vi "Updating Existing Tree from XML.vi"() -> ()   [LabVIEW 2017, in "Tree API.lvlib" / "Tree.lvclass"]
uses:
  Tree.lvclass
  API/Set Attributes Tree Data.vi
  Data Types/Float/To Float Tree Data.vi
  Data Types/Float/Flt.lvclass
  Data Types/Bool/To Bool Tree Data.vi
  Data Types/Bool/Bool.lvclass
panel:
  in  "Setpoint 2":dbl=2.0 format="%#_13g"
  in  "Setpoint 1":dbl=-1.0 format="%#_13g"
  in  "Run HW":bool=TRUE
  in  "Enable CFG":bool
  out "XML On RT":string="<Received_Configuration>\n<Enable_CFG Type=\"Bool\">\r\nFALSE\r\n</Enable_CFG>\r\n<Run_HW Type=\"Bool\">\r\nTRUE\r\n</Run_HW>\r\n<Setpoint_1 Type=\"Flt\">\r\n-1\r\n</Setpoint_1>\r\n<Setpoint_2 Type=\"Flt\">\r\n2\r\n</Setpoint_2>\n\n</Received_Configuration>"
  out "XML On Host":string="<Configuration>\n<Enable_CFG Type=\"Bool\">\r\nFALSE\r\n</Enable_CFG>\r\n<Run_HW Type=\"Bool\">\r\nTRUE\r\n</Run_HW>\r\n<Setpoint_1 Type=\"Flt\">\r\n-1\r\n</Setpoint_1>\r\n<Setpoint_2 Type=\"Flt\">\r\n2\r\n</Setpoint_2>\n\n</Configuration>"
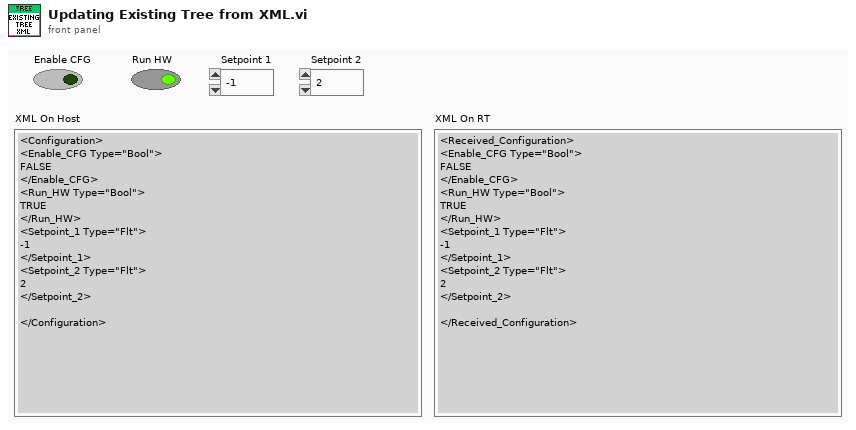
[diagram p1: front panel]
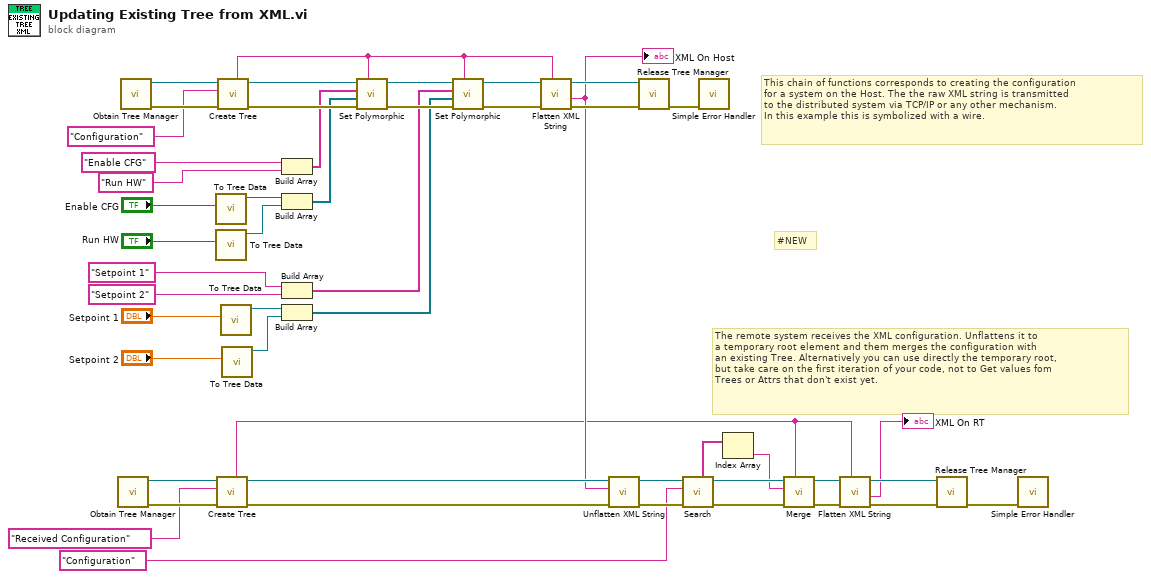
[diagram p0: block diagram]
diagram:
  # "#NEW"
  # "The remote system receives the XML configuration. Unflattens it to\na temporary root element and them merges the configuration with\nan existing Tree. Alternatively you can use directly the temporary root,\nbut take care on the first iteration of your code, not to Get values fom \nTrees or Attrs that don't exist yet."
  # "This chain of functions corresponds to creating the configuration\nfor a system on the Host. The the raw XML string is transmitted\nto the distributed system via TCP/IP or any other mechanism.\nIn this example this is symbolized with a wire."
  n1 = call "Obtain Tree Manager.vi"() -> ("Error Out"=w24:errorcluster, "Tree"=w25:refnum<data-value>)  [unwired: 10 in]
  n2 = call "Obtain Tree Manager.vi"() -> ("Error Out"=w48:errorcluster, "Tree"=w49:refnum<data-value>)  [unwired: 10 in]
  n3 = call-poly "To Tree Data.vi"("Boolean"="Enable CFG") -> ("Bool Tree Data"=w41:refnum<class "Bool.lvclass">)  [unwired: 10 in]
  n4 = call-poly "To Tree Data.vi"("Boolean"="Run HW") -> ("Bool Tree Data"=w5:refnum<class "Bool.lvclass">)  [unwired: 10 in]
  n5 = call "Create Tree.vi"("Error In"=w24, "Name"="Received Configuration", "Tree Manager"=w25) -> ("Error Out"=w21:errorcluster, "Tree Manager"=w22:refnum<data-value>, "Unique ID"=w10:string)  [unwired: 6 in]
  n6 = call "Create Tree.vi"("Error In"=w48, "Name"="Configuration", "Tree Manager"=w49) -> ("Error Out"=w44:errorcluster, "Tree Manager"=w45:refnum<data-value>, "Unique ID"=w28:string)  [unwired: 6 in]
  n7 = call-poly "To Tree Data.vi"("Float"="Setpoint 1") -> ("Float Tree Data"=w35:refnum<class "Flt.lvclass">)  [unwired: 10 in]
  n8 = call-poly "To Tree Data.vi"("Float"="Setpoint 2") -> ("Float Tree Data"=w4:refnum<class "Flt.lvclass">)  [unwired: 10 in]
  n9 = Build Array("Enable CFG" ("Attribute Name"), "Run HW" ("Attribute Name")) -> (w39:string[])
  n10 = Build Array(w41, w5) -> (w40:refnum<class "Bool.lvclass">[])
  n11 = Build Array("Setpoint 1" ("Attribute Name"), "Setpoint 2" ("Attribute Name")) -> (w32:string[])
  n12 = Build Array(w35, w4) -> (w31:refnum<class "Flt.lvclass">[])
  n13 = call-poly "Set Polymorphic.vi"("Tree ID"=w28, "Error In"=w44, "Attributes Values"=w40, "Attributes Names"=w39, "Tree Manager"=w45) -> ("Error Out"=w37:errorcluster, "Tree Manager"=w38:refnum<data-value>)  [unwired: 4 in, 1 out]
  n14 = call-poly "Set Polymorphic.vi"("Tree ID"=w28, "Error In"=w37, "Attributes Values"=w31, "Attributes Names"=w32, "Tree Manager"=w38) -> ("Error Out"=w29:errorcluster, "Tree Manager"=w30:refnum<data-value>)  [unwired: 4 in, 1 out]
  n15 = call "Flatten XML String.vi"("Root ID"=w28, "Error In"=w29, "Tree"=w30) -> ("Error Out"=w26:errorcluster, "XML String"=w20:string, "Tree"=w27:refnum<data-value>)  [unwired: 6 in]
  "XML On Host" <- w20
  n16 = call "Unflatten XML String.vi"("Error In"=w21, "XML String"=w20, "Tree"=w22) -> ("Error Out"=w18:errorcluster, "Tree"=w19:refnum<data-value>)  [unwired: 7 in]
  n17 = call "Release Tree Manager.vi"("Error In"=w26, "Tree"=w27) -> ("Error Out"=w1:errorcluster)  [unwired: 9 in]
  n18 = call "Search.vi"("Error In"=w18, "Name or Tree Path"="Configuration" ("Name"), "Tree Manager"=w19) -> ("Error Out"=w14:errorcluster, "Tree Manager"=w15:refnum<data-value>, "IDs"=w16:string[])  [unwired: 6 in]
  n19 = call <vilib>:"Simple Error Handler.vi"("error in (no error)"=w1) -> ()  [unwired: 4 in, 5 out]
  n20 = Index Array(array=w16) -> (element=w13:string)  [unwired: 1 in]
  n21 = call "Merge.vi"("Target Tree ID"=w10, "Error In"=w14, "Source Tree ID"=w13, "Tree Manager"=w15) -> ("Error Out"=w11:errorcluster, "Tree Manager"=w12:refnum<data-value>)  [unwired: 6 in]
  n22 = call "Flatten XML String.vi"("Root ID"=w10, "Error In"=w11, "Tree"=w12) -> ("Error Out"=w8:errorcluster, "XML String"=→"XML On RT":string, "Tree"=w9:refnum<data-value>)  [unwired: 6 in]
  n23 = call "Release Tree Manager.vi"("Error In"=w8, "Tree"=w9) -> ("Error Out"=w2:errorcluster)  [unwired: 9 in]
  n24 = call <vilib>:"Simple Error Handler.vi"("error in (no error)"=w2) -> ()  [unwired: 4 in, 5 out]
